vi "Read Product Name.vi"(8 "error in (no error)":errorcluster, 11 "ACM 4509 Cal Standard in":refnum<class "Cal Standard.lvclass">) -> (0 "error out":errorcluster, 2 "Product Name":string, 3 "ACM 4509 Cal Standard out":refnum<class "Cal Standard.lvclass">)   [LabVIEW 2023, in "ACM 4509 Cal Standard.lvlib" / "Cal Standard.lvclass"]
uses:
  Cal Standard.lvclass
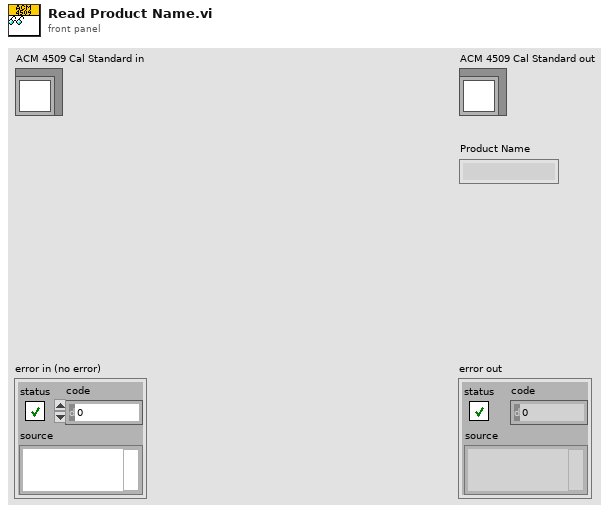
[diagram p1: front panel]
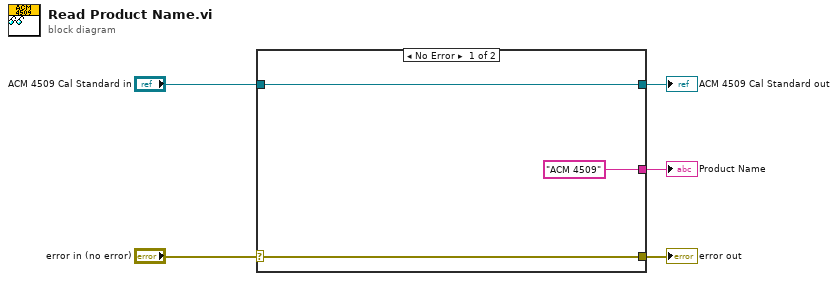
[diagram p0: block diagram]
diagram:
  n1 = case shown="No Error" "error in (no error)" {
    selector: "error in (no error)" -> [w8 w9]
    tunnel: [w8 w9] -> w4
    tunnel: [w7 w10] -> w2
    tunnel: "ACM 4509 Cal Standard in" -> [w7 w10]
    tunnel: ["ACM 4509" ("Product Name") _] -> w1
    frame No Error {
    }
    frame Error {
    }
  }
  "error out" <- w4
  "ACM 4509 Cal Standard out" <- w2
  "Product Name" <- w1
